vi "Bag Remover Wash.vi"(11 "IO":T1) -> (3 "bt_Node out":refnum<class "bt_Node.lvclass">)   [LabVIEW 2021, in "Car Wash Support.lvlib"]
uses:
  Car Wash Support.lvlib
  IO Refs.ctl
  <vilib>/TSA/Event Log/Event_TextLog/Event_TextLog.lvclass
  <vilib>/TSA/Abstract Data Classes/Abs_Types/Boolean/Abs_Boolean.lvclass
  <vilib>/TSA/Abstract Data Classes/Abs_Types/I32 Integer/Abs_I32 Integer.lvclass
  <vilib>/TSA/Abstract Data Classes/Abs_Types/Double Float/Abs_Double Float.lvclass
  Wash Indicators.ctl
  Wash Options.ctl
  Support/Nodes/abs_Node/bt_Node.lvclass
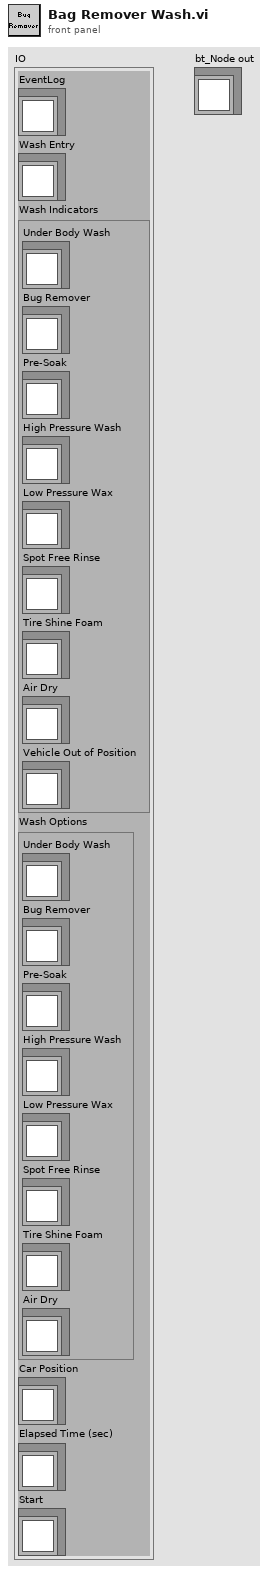
[diagram p1: front panel]
types:
  T1 = typedef "Car Wash Support.lvlib/IO Refs.ctl" = cluster{"EventLog":refnum<class "Event_TextLog.lvclass">, "Wash Entry":refnum<class "Abs_Boolean.lvclass">, "Wash Indicators":T2, "Wash Options":T3, "Car Position":refnum<class "Abs_I32 Integer.lvclass">, "Elapsed Time (sec)":refnum<class "Abs_Double Float.lvclass">, "Start":refnum<class "Abs_Boolean.lvclass">}
  T2 = typedef "Car Wash Support.lvlib/Wash Indicators.ctl" = cluster{"Under Body Wash":refnum<class "Abs_Boolean.lvclass">, "Bug Remover":refnum<class "Abs_Boolean.lvclass">, "Pre-Soak":refnum<class "Abs_Boolean.lvclass">, "High Pressure Wash":refnum<class "Abs_Boolean.lvclass">, "Low Pressure Wax":refnum<class "Abs_Boolean.lvclass">, "Spot Free Rinse":refnum<class "Abs_Boolean.lvclass">, "Tire Shine Foam":refnum<class "Abs_Boolean.lvclass">, "Air Dry":refnum<class "Abs_Boolean.lvclass">, "Vehicle Out of Position":refnum<class "Abs_Boolean.lvclass">}
  T3 = typedef "Car Wash Support.lvlib/Wash Options.ctl" = cluster{"Under Body Wash":refnum<class "Abs_Boolean.lvclass">, "Bug Remover":refnum<class "Abs_Boolean.lvclass">, "Pre-Soak":refnum<class "Abs_Boolean.lvclass">, "High Pressure Wash":refnum<class "Abs_Boolean.lvclass">, "Low Pressure Wax":refnum<class "Abs_Boolean.lvclass">, "Spot Free Rinse":refnum<class "Abs_Boolean.lvclass">, "Tire Shine Foam":refnum<class "Abs_Boolean.lvclass">, "Air Dry":refnum<class "Abs_Boolean.lvclass">}
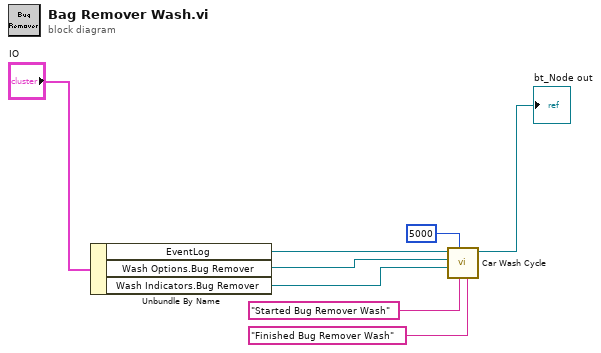
[diagram p0: block diagram]
diagram:
  n1 = Unbundle By Name("IO") -> ("EventLog"=w3:refnum<class "Event_TextLog.lvclass">, "Wash Options.Bug Remover"=w4:refnum<class "Abs_Boolean.lvclass">, "Wash Indicators.Bug Remover"=w5:refnum<class "Abs_Boolean.lvclass">)
  n2 = call "Car Wash Cycle.vi"("Finish Message"="Finished Bug Remover Wash", "Start Message"="Started Bug Remover Wash", "Time (ms)"=u32 5000, "Indicator"=w5, "Option"=w4, "EventLog"=w3) -> ("bt_Node out"=→"bt_Node out":refnum<class "bt_Node.lvclass">)  [unwired: 5 in]
